vi "PoseAndTargeting.vi"() -> ()   [LabVIEW 2019]
doc: "This VI manages the robot's pose and targetting information. Data from the IMU, swerve drive encoders, swerve azimuth encoders, LimeLight, and LIDAR are fused together to estimate these values. Supports pose resets on boot, from the Autonomous Sequencer, and on command from the FRC 4265 Dashboard."
uses:
  dsinstructions.vi
  sensors.vi
  dsdata.vi
  outputs.vi
panel:
  out "Y Position (in)":dbl
  out "X Position (in)":dbl
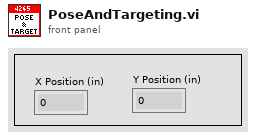
[diagram p1: front panel]
types:
  T1 = enum16{"Center", "North", "NorthWest", "West", "SouthWest", "South", "SouthEast", "East", "NorthEast"}
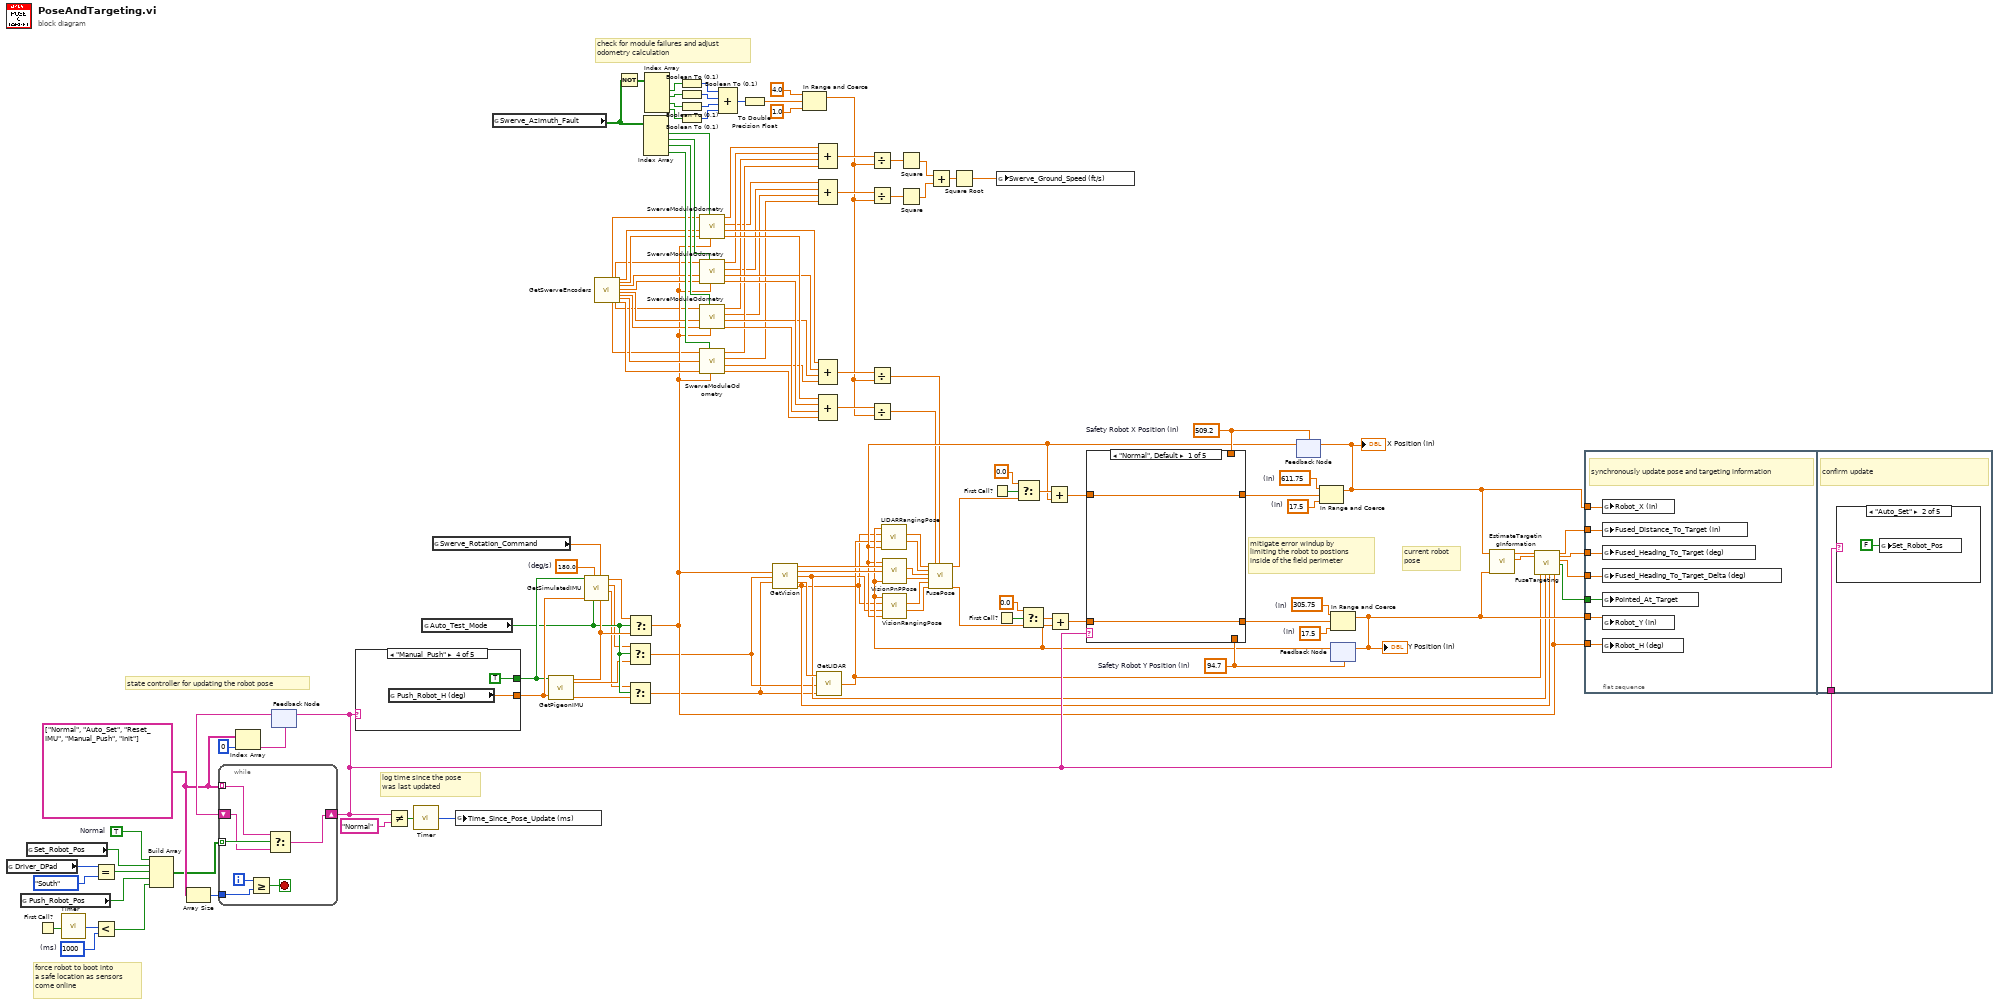
[diagram p0: block diagram]
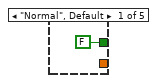
[diagram p6: hidden frame]
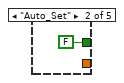
[diagram p7: hidden frame]
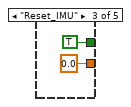
[diagram p8: hidden frame]
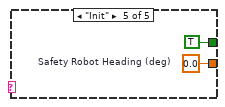
[diagram p9: hidden frame]
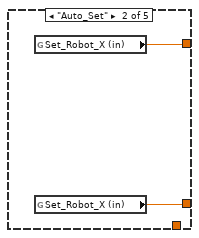
[diagram p10: hidden frame]
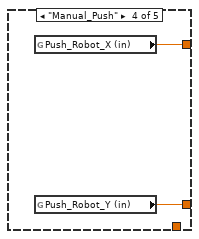
[diagram p12: hidden frame]
diagram:
  w73 = 180.0  # (deg/s)
  w77 = u32 1000  # (ms)
  w95 = string[] ["Normal", "Auto_Set", "Reset_IMU", "Manual_Push", "Init"] ("State Names")
  w94 = TRUE  # Normal
  w104 = 305.75  # (in)
  w105 = 17.5  # (in)
  w109 = 611.75  # (in)
  w110 = 17.5  # (in)
  w82 = 509.2  # Safety Robot X Position (in)
  w81 = 94.7  # Safety Robot Y Position (in)
  # "force robot to boot into\na safe location as sensors\ncome online"
  # "log time since the pose\nwas last updated"
  # "state controller for updating the robot pose"
  # "current robot\npose"
  # "mitigate error windup by\nlimiting the robot to postions\ninside of the field perimeter"
  # "check for module failures and adjust\nodometry calculation"
  n1 = global read "dsinstructions.vi" "Driver_DPad"() -> (w112:T1)
  n2 = global read "sensors.vi" "Push_Robot_Pos"() -> (w96:bool)
  n3 = global read "sensors.vi" "Set_Robot_Pos"() -> (w72:bool)
  n4 = First Call?() -> (First Call?: T/F=w80:bool)
  n5 = call "Timer.vi"("Reset Timer"=w80) -> ("Time (ms)"=w79:u32)
  n6 = Equal?(x=w112, y=T1."South") -> (x = y?=w71:bool)
  n7 = Less?(x=w79, y=w77) -> (x < y?=w78:bool)
  n8 = Build Array(w94, w72, w71, w96, w78) -> (w93:bool[])
  n9 = Array Size(array=w95) -> (size(s)=w97:i32)
  n10 = Index Array(array=w95, index=0) -> (element=w99:string)
  n11 = feedback #1(w99) -> (w98:string)
  n12 = while {
    tunnel: w93 -> [w140] mode=indexing
    tunnel: w95 -> [w138] mode=indexing
    shift-right: [w137] -> w86
    shift-left: w98 -> [w139]
    tunnel: w97 -> [w135]
    i -> [w136]
    stop <- w134 stop-if-true
    n13 = Greater Or Equal?(x=w136, y=w135) -> (x >= y?=w134:bool)
    n14 = Select(t=w138, s=w140, f=w139) -> (s? t:f=w137:string)
  }
  n15 = feedback-in #1(w86) -> ()
  n16 = case shown="\"Manual_Push\"" w86 {
    tunnel: [_ _ 0.0 ("Push_Robot_H (deg)") w146 w147] -> w76
    tunnel: [FALSE FALSE TRUE TRUE TRUE] -> w75
    frame "Normal", Default {
    }
    frame "Auto_Set" {
    }
    frame "Reset_IMU" {
    }
    frame "Manual_Push" {
      n17 = global read "sensors.vi" "Push_Robot_H (deg)"() -> (w146:dbl)
    }
    frame "Init" {
      w147 = 0.0  # Safety Robot Heading (deg)
    }
  }
  n18 = Not Equal?(x=w86, y="Normal") -> (x != y?=w85:bool)
  n19 = call "Timer.vi"("Reset Timer"=w85) -> ("Time (ms)"=w83:u32)
  n20 = global read "dsdata.vi" "Auto_Test_Mode"() -> (w33:bool)
  n21 = global read "outputs.vi" "Swerve_Rotation_Command"() -> (w74:dbl)
  n22 = global write "sensors.vi" "Time_Since_Pose_Update (ms)"(w83) -> ()
  n23 = global read "sensors.vi" "Swerve_Azimuth_Fault"() -> (w127:bool[])
  n24 = call "GetPigeonIMU.vi"("Reset Yaw (deg)"=w76, "Reset Yaw"=w75) -> ("Roll (deg)"=w29:dbl, "Pitch (deg)"=w31:dbl, "Yaw (deg)"=w34:dbl)  [unwired: 7 in]
  n25 = call "GetSimulatedIMU.vi"("Real IMU Yaw (deg)"=w34, "Rotation Command"=w74, "Auto Test Mode"=w33, "Max Simulated Rotation Speed (deg/s)"=w73, "Reset Yaw (deg)"=w76, "Reset Yaw"=w75) -> ("Simulated Roll (deg)"=w30:dbl, "Simulated Pitch (deg)"=w32:dbl, "Simulated Yaw (deg)"=w35:dbl)  [unwired: 3 in]
  n26 = call "GetSwerveEncoders.vi"() -> ("Swerve 0 Velocity (ft/s)"=w4:dbl, "Swerve 3 Velocity (ft/s)"=w1:dbl, "Swerve 1 Velocity (ft/s)"=w3:dbl, "Swerve 2 Velocity (ft/s)"=w2:dbl, "Swerve 0 Azimuth Position (deg)"=w70:dbl, "Swerve 0 Distance (in)"=w63:dbl, "Swerve 1 Azimuth Position (deg)"=w69:dbl, "Swerve 1 Distance (in)"=w68:dbl, "Swerve 2 Azimuth Position (deg)"=w67:dbl, "Swerve 2 Distance (in)"=w66:dbl, "Swerve 3 Azimuth Position (deg)"=w65:dbl, "Swerve 3 Distance (in)"=w64:dbl)  [unwired: 16 in]
  n27 = Not(x=w127) -> (.not. x?=w126:bool[])
  n28 = Select(t=w32, s=w33, f=w31) -> (s? t:f=w27:dbl)
  n29 = Select(t=w30, s=w33, f=w29) -> (s? t:f=w26:dbl)
  n30 = Select(t=w35, s=w33, f=w34) -> (s? t:f=w28:dbl)
  n31 = Index Array(array=w127) -> (element #1=w116:bool, element #2=w115:bool, element #3=w114:bool, element #4=w113:bool)  [unwired: 4 in]
  n32 = Index Array(array=w126) -> (element #1=w125:bool, element #2=w124:bool, element #3=w123:bool, element #4=w122:bool)  [unwired: 4 in]
  n33 = Boolean To (0,1)(Boolean=w125) -> (0, 1=w121:i16)
  n34 = Boolean To (0,1)(Boolean=w124) -> (0, 1=w120:i16)
  n35 = Boolean To (0,1)(Boolean=w123) -> (0, 1=w119:i16)
  n36 = Boolean To (0,1)(Boolean=w122) -> (0, 1=w118:i16)
  n37 = call "SwerveModuleOdometry.vi"("Robot Heading(deg)"=w28, "Module Fault"=w116, "Wheel Distance (in)"=w63, "Wheel Azimuth (deg)"=w70, "Velocity (ft/s)"=w4) -> ("Delta Y (in)"=w128:dbl, "Delta X (in)"=w25:dbl, "Velocity Y (ft/s)"=w17:dbl, "Velocity X (ft/s)"=w21:dbl)  [unwired: 1 in]
  n38 = call "SwerveModuleOdometry.vi"("Robot Heading(deg)"=w28, "Module Fault"=w115, "Wheel Distance (in)"=w68, "Wheel Azimuth (deg)"=w69, "Velocity (ft/s)"=w3) -> ("Delta Y (in)"=w129:dbl, "Delta X (in)"=w24:dbl, "Velocity Y (ft/s)"=w16:dbl, "Velocity X (ft/s)"=w20:dbl)  [unwired: 1 in]
  n39 = call "SwerveModuleOdometry.vi"("Robot Heading(deg)"=w28, "Module Fault"=w114, "Wheel Distance (in)"=w66, "Wheel Azimuth (deg)"=w67, "Velocity (ft/s)"=w2) -> ("Delta Y (in)"=w130:dbl, "Delta X (in)"=w23:dbl, "Velocity Y (ft/s)"=w15:dbl, "Velocity X (ft/s)"=w19:dbl)  [unwired: 1 in]
  n40 = call "SwerveModuleOdometry.vi"("Robot Heading(deg)"=w28, "Module Fault"=w113, "Wheel Distance (in)"=w64, "Wheel Azimuth (deg)"=w65, "Velocity (ft/s)"=w1) -> ("Delta Y (in)"=w131:dbl, "Delta X (in)"=w22:dbl, "Velocity Y (ft/s)"=w14:dbl, "Velocity X (ft/s)"=w18:dbl)  [unwired: 1 in]
  n41 = Compound Arithmetic op=ADD(w121, w120, w119, w118) -> (w117:i16)
  n42 = To Double Precision Float(number=w117) -> (double precision float=w58:dbl)
  n43 = call "GetVision.vi"("Robot_H (deg)"=w28, "Pitch (deg)"=w27, "Roll (deg)"=w26) -> ("LimeLight Raw Z (in)"=w62:dbl, "LimeLight Raw X (in)"=w61:dbl, "LimeLight Distance to Target (in)"=w41:dbl, "LimeLight Raw Horizontal Offset (deg)"=w43:dbl, "LimeLight Heading to Target (deg)"=w36:dbl)  [unwired: 8 in]
  n44 = In Range and Coerce(upper limit=4.0, x=w58, lower limit=1.0) -> (coerced(x)=w11:dbl)  [unwired: 1 out]
  n45 = call "GetLIDAR.vi"("Roll (deg)"=w26, "Pitch (deg)"=w27, "Raw Horizontal Offset (in)"=w43) -> ("LIDAR Distance to Target (in)"=w42:dbl)
  n46 = Compound Arithmetic op=ADD(w21, w20, w19, w18) -> (w13:dbl)
  n47 = Compound Arithmetic op=ADD(w17, w16, w15, w14) -> (w12:dbl)
  n48 = Compound Arithmetic op=ADD(w25, w24, w23, w22) -> (w133:dbl)
  n49 = Compound Arithmetic op=ADD(w128, w129, w130, w131) -> (w132:dbl)
  n50 = Divide(x=w13, y=w11) -> (x/y=w7:dbl)
  n51 = Divide(x=w12, y=w11) -> (x/y=w6:dbl)
  n52 = Divide(x=w133, y=w11) -> (x/y=w53:dbl)
  n53 = Divide(x=w132, y=w11) -> (x/y=w52:dbl)
  n54 = Square(x=w7) -> (x^2=w9:dbl)
  n55 = Square(x=w6) -> (x^2=w10:dbl)
  n56 = Add(x=w9, y=w10) -> (x+y=w8:dbl)
  n57 = Square Root(x=w8) -> (sqrt(x)=w5:dbl)
  n58 = First Call?() -> (First Call?: T/F=w107:bool)
  n59 = First Call?() -> (First Call?: T/F=w102:bool)
  n60 = global write "sensors.vi" "Swerve_Ground_Speed (ft/s)"(w5) -> ()
  n61 = feedback #2(w82) -> (w59:dbl)
  n62 = feedback #3(w81) -> (w60:dbl)
  n63 = call "LIDARRangingPose.vi"("Previous X Position (in)"=w59, "Distance to Target (in)"=w42, "Heading to Target (deg)"=w36, "Previous Y Position (in)"=w60) -> ("Delta Y (in)"=w50:dbl, "Delta X (in)"=w51:dbl)  [unwired: 6 in]
  n64 = call "VisionPnPPose.vi"("Previous Y Estimate (in)"=w60, "LimeLight Raw X (in)"=w61, "LimeLight Raw Z (in)"=w62, "Previous X Estimate (in)"=w59) -> ("deltaY (in)"=w48:dbl, "deltaX (in)"=w49:dbl)  [unwired: 6 in]
  n65 = call "VisionRangingPose.vi"("Previous X Position (in)"=w59, "Distance to Target (in)"=w41, "Heading to Target (deg)"=w36, "Previous Y Position (in)"=w60) -> ("Delta Y (in)"=w46:dbl, "Delta X (in)"=w47:dbl)  [unwired: 6 in]
  n66 = call "FusePose.vi"("LIDAR range deltaX"=w51, "LIDAR range deltaY"=w50, "LimeLight PnP deltaX"=w49, "LimeLight PnP deltaY"=w48, "LimeLight range deltaX"=w47, "LimeLight range deltaY"=w46, "Odometry deltaY"=w52, "Odometry deltaX"=w53) -> ("Fused deltaX"=w55:dbl, "Fused deltaY"=w54:dbl)  [unwired: 10 in]
  n67 = Select(t=0.0, s=w107, f=w55) -> (s? t:f=w108:dbl)
  n68 = Select(t=0.0, s=w102, f=w54) -> (s? t:f=w103:dbl)
  n69 = Add(x=w108, y=w59) -> (x+y=w92:dbl)
  n70 = Add(x=w103, y=w60) -> (x+y=w90:dbl)
  n71 = case shown="\"Normal\", Default" w86 {
    tunnel: w92 -> [w150 _ w154 _ _]
    tunnel: [w150 w152 w154 w156 w158] -> w91
    tunnel: w90 -> [w149 _ w153 _ _]
    tunnel: [w149 w151 w153 w155 w157] -> w89
    tunnel: w82 -> [_ _ _ _ w158]
    tunnel: w81 -> [_ _ _ _ w157]
    frame "Normal", Default {
    }
    frame "Auto_Set" {
      n72 = global read "sensors.vi" "Set_Robot_X (in)"() -> (w152:dbl)
      n73 = global read "sensors.vi" "Set_Robot_X (in)"() -> (w151:dbl)
    }
    frame "Reset_IMU" {
    }
    frame "Manual_Push" {
      n74 = global read "sensors.vi" "Push_Robot_X (in)"() -> (w156:dbl)
      n75 = global read "sensors.vi" "Push_Robot_Y (in)"() -> (w155:dbl)
    }
    frame "Init" {
    }
  }
  n76 = In Range and Coerce(upper limit=w109, x=w91, lower limit=w110) -> (coerced(x)=w88:dbl)  [unwired: 1 out]
  "X Position (in)" <- w88
  n77 = feedback-in #2(w88) -> ()
  n78 = In Range and Coerce(upper limit=w104, x=w89, lower limit=w105) -> (coerced(x)=w87:dbl)  [unwired: 1 out]
  "Y Position (in)" <- w87
  n79 = feedback-in #3(w87) -> ()
  n80 = call "EstimateTargetingInformation.vi"("Robot Y (in)"=w87, "Robot X (in)"=w88) -> ("Estimated Robot Heading to Target (deg)"=w44:dbl, "Estimated Distance to Target (in)"=w45:dbl)  [unwired: 7 in]
  n81 = call "FuseTargeting.vi"("Estimated Distance to Target (in)"=w45, "Estimated Heading to Target (deg)"=w44, "LIDAR Distance to Target (in)"=w42, "LimeLight Distance to Target (in)"=w41, "LimeLight Heading to Target (deg)"=w36, "Robot_H (deg)"=w28) -> ("Fused Distance to Target (in)"=w40:dbl, "Fused Heading to Target (deg)"=w39:dbl, "Fused Heading to Target Delta (deg)"=w38:dbl, "Pointed at Target"=w37:bool)  [unwired: 10 in]
  n82 = flat-sequence {
    tunnel: w88 -> [w165]
    tunnel: w87 -> [w164]
    tunnel: w28 -> [w163]
    tunnel: w40 -> [w162]
    tunnel: w39 -> [w161]
    tunnel: w38 -> [w160]
    tunnel: w37 -> [w159]
    tunnel: w86 -> [w166]
    frame #0 {
      # "synchronously update pose and targeting information"
      n83 = global write "sensors.vi" "Robot_X (in)"(w165) -> ()
      n84 = global write "sensors.vi" "Fused_Distance_To_Target (in)"(w162) -> ()
      n85 = global write "sensors.vi" "Fused_Heading_To_Target (deg)"(w161) -> ()
      n86 = global write "sensors.vi" "Fused_Heading_To_Target_Delta (deg)"(w160) -> ()
      n87 = global write "sensors.vi" "Pointed_At_Target"(w159) -> ()
      n88 = global write "sensors.vi" "Robot_Y (in)"(w164) -> ()
      n89 = global write "sensors.vi" "Robot_H (deg)"(w163) -> ()
    }
    frame #1 {
      # "confirm update"
      n90 = case shown="\"Auto_Set\"" w166 {
        frame "Normal", Default {
        }
        frame "Auto_Set" {
          n91 = global write "sensors.vi" "Set_Robot_Pos"(FALSE ("Set_Robot_Pos")) -> ()
        }
        frame "Reset_IMU" {
        }
        frame "Manual_Push" {
        }
        frame "Init" {
        }
      }
    }
  }
